vi "IMULoop.vi"(6 "I2CDevRef 2":T9={"DevStatus"={"status"=FALSE, "code"=0, "source"=""}, "Device Address"=0, "Handle"=0, "I2C Bus"=enum."Invalid"} {"Device Address" format="%.0x"}, 8 "AccelerometerDevRef":T1={"DevStatus"={"status"=FALSE, "code"=0, "source"=""}, "Scaling"={"Gain (VoltsPerG)"=0.0, "Center Voltage"=0.0}, "Analog Channels"={"X-Axis"=enum."Invalid", "Y-Axis"=enum."Invalid", "Z-Axis"=enum."Invalid"}, "I2C Bus"=enum."Invalid", "SPI Bus"=enum."Invalid", "Accel Range"=0, "ADXL345 Axes"={"X-Axis"=FALSE, "Y-Axis"=FALSE, "Z-Axis"=FALSE}, "Handle"=0, "Device Address"=0, "Accel Type"=enum."Analog"} {"Device Address" format="%.0x"; "Accel Range" items=["+/- 2 g", "+/- 4 g", "+/- 8 g", "+/- 16 g"]}) -> ()   [LabVIEW 2015]
uses:
  <vilib>/Rock Robotics/WPI/I2C/WPI_I2CDevRef.ctl
  <vilib>/Rock Robotics/SystemInterfaces/i2clib/i2c_bus.ctl
  <vilib>/Rock Robotics/WPI/Accelerometer/WPI_AccelerometerDevRef.ctl
  <vilib>/Rock Robotics/WPI/Accelerometer/WPI_AccelerometerScaling.ctl
  <vilib>/Rock Robotics/WPI/Accelerometer/WPI_AccelerometerAnalogChannels.ctl
  <vilib>/Rock Robotics/SystemInterfaces/AI/FPGA_AIChannel.ctl
  <vilib>/Rock Robotics/SystemInterfaces/spilib/spi_bus.ctl
  <vilib>/Rock Robotics/WPI/Accelerometer/ADXL345 Range.ctl
  <vilib>/Rock Robotics/WPI/Accelerometer/WPI_AccelerometerADXL345 Axes.ctl
  Common Code/IMU Data.ctl
  navX-MXP Library/COMMON/TypeDefs/Value TypeDefs/navX NAVX_CAL_STATUS.ctl
  navX-MXP Library/COMMON/TypeDefs/Value TypeDefs/navX NAVX_OP_STATUS.ctl
  Robot Global Data.vi
  <vilib>/Platform/TimedLoop/XDataNode/XDataNode.xnode
  <vilib>/Platform/TimedLoop/XDataNode/nitl_modes.ctl
  <vilib>/Platform/TimedLoop/XDataNode/XDNodeRunTimeDep.lvlib
  <vilib>/Platform/TimedLoop/XDataNode/wakeup.ctl
  <vilib>/Platform/TimedLoop/XDataNode/timing_clust.ctl
  navX-MXP Library/navX-MXP IMU.lvlib
panel:
  # "ADXL345"
  # "Analog"
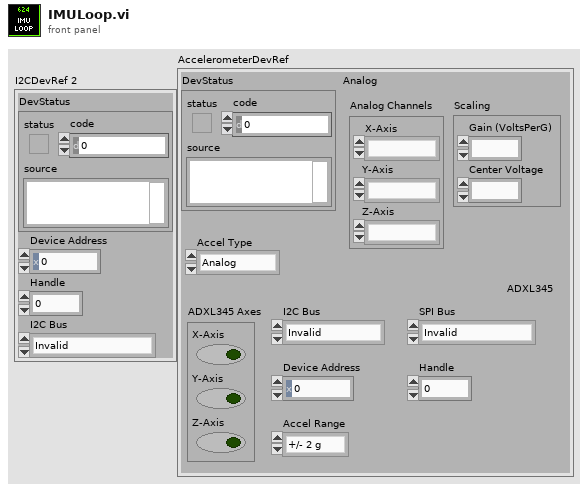
[diagram p1: front panel]
types:
  T1 = typedef "WPI_AccelerometerDevRef.ctl" = cluster{"DevStatus":errorcluster, "Scaling":T2, "Analog Channels":T3, "I2C Bus":T5, "SPI Bus":T6, "Accel Range":T7, "ADXL345 Axes":T8, "Handle":i32, "Device Address":u8, "Accel Type":enum16{"Analog", "ADXL345 I2C", "ADXL345 SPI", "Internal"}}
  T2 = typedef "WPI_AccelerometerScaling.ctl" = cluster{"Gain (VoltsPerG)":dbl, "Center Voltage":dbl}
  T3 = typedef "WPI_AccelerometerAnalogChannels.ctl" = cluster{"X-Axis":T4, "Y-Axis":T4, "Z-Axis":T4}
  T4 = typedef "FPGA_AIChannel.ctl" = enum8{"AI 0", "AI 1", "AI 2", "AI 3", "AI MXP 0", "AI MXP 1", "AI MXP 2", "AI MXP 3", "Invalid"}
  T5 = typedef "i2c_bus.ctl" = enum16{"I2C On-Board", "I2C MXP", "Invalid"}
  T6 = typedef "spi_bus.ctl" = enum16{"SPI On-Board, CS0", "SPI On-Board, CS1", "SPI On-Board, CS2", "SPI On-Board, CS3", "SPI MXP", "Invalid"}
  T7 = typedef "ADXL345 Range.ctl" = u8
  T8 = typedef "WPI_AccelerometerADXL345 Axes.ctl" = cluster{"X-Axis":bool, "Y-Axis":bool, "Z-Axis":bool}
  T9 = typedef "WPI_I2CDevRef.ctl" = cluster{"DevStatus":errorcluster, "Device Address":u8, "Handle":i32, "I2C Bus":T5}
  T10 = typedef "IMU Data.ctl" = cluster{"Pitch":sgl, "Roll":sgl, "Yaw":sgl, "Data Valid?":bool, "Temp":sgl, "MOVING":bool, "NAVX_CAL_STATUS":T11, "NAVX_OP_STATUS":T12, "YAW_STABLE":bool, "Accel X":sgl, "Accel Y":sgl, "Accel Z":sgl, "Accel Magnitude":sgl, "Pitch Rate":sgl, "Roll Rate":sgl, "Yaw Rate":sgl, "NavX Opened?":bool}
  T11 = typedef "navX-MXP IMU.lvlib/navX NAVX_CAL_STATUS.ctl" = u8
  T12 = typedef "navX-MXP IMU.lvlib/navX NAVX_OP_STATUS.ctl" = u8
  T13 = typedef "XDNodeRunTimeDep.lvlib/timing_clust.ctl" = cluster{"Expected End [f-1]":u64, "Actual End [f-1]":u64, "Finished Late? [f-1]":bool, "Expected End [i-1]":u64, "Actual End [i-1]":u64, "Finished Late? [i-1]":bool, "Expected Start [i]":u64, "Actual Start [i]":u64, "Expected Start [f]":u64, "Actual Start [f]":u64, "Source Name":string, "Structure Name":string, "Period":i64, "Deadline":i64, "Offset":i64, "Start":i64, "Priority":i32, "Timeout":i32, "Mode":T14, "Wakeup Reason":T15, "Error":errorcluster, "Source Type":string, "Secondary Source Type":string, "Global End Time":u64, "Global Start Time":u64, "Frame Duration":u64, "Iteration Duration":u64, "Assigned CPU":i32, "I/O Scan Engine Mode":u32}
  T14 = typedef "XDNodeRunTimeDep.lvlib/nitl_modes.ctl" = enum32{"No Change", "Process missed periods, maintain original phase", "Discard missed periods, maintain original phase", "Process missed periods, ignore original phase", "Discard missed periods, ignore original phase"}
  T15 = typedef "XDNodeRunTimeDep.lvlib/wakeup.ctl" = enum32{"Normal", "Aborted", "Asynchronous wakeup", "Timing source error", "Timed loop error", "Timeout"}
  T16 = cluster{"X-Axis":dbl, "Y-Axis":dbl, "Z-Axis":dbl}
  T17 = typedef "navX-MXP IMU.lvlib/navX Device TypeDef.ctl" = cluster{"navX Interface Protocol":T18, "navX Interface Protocol TypeDefs":cluster{"SPIDevRef":T19, "I2CDevRef":T9}, "navX System Information":cluster{"Board Information":T20, "Status":T21, "Offsets":T23}, "navX Common Information":cluster{"Update Rate (4Hz-60Hz)":T24, "refnum name":string, "error":errorcluster}}
  T18 = typedef "navX-MXP IMU.lvlib/navX Interface Protocol.ctl" = enum16{"SPI", "I2C"}
  T19 = typedef "WPI_SPIDevRef.ctl" = cluster{"DevStatus":errorcluster, "Handle":i32, "SPI Bus":T6}
  T20 = typedef "navX-MXP IMU.lvlib/navX Board Information.ctl" = cluster{"WhoAmI (50 | 0x32)":u8, "Board Revision":u8, "Firmware Major Version":u8, "Firmware Minor Version":u8}
  T21 = typedef "navX-MXP IMU.lvlib/navX Status Data.ctl" = cluster{"Update Rate Hz":u8, "Accelerometer Full-Scale Range":u8, "Gyro Full-Scale Range":u16, "NAVX_OP_STATUS":T12, "NAVX_CAL_STATUS":T11, "NAVX_SELFTEST_STATUS":u8, "NAVX_SENSOR_STATUS":T22}
  T22 = typedef "navX-MXP IMU.lvlib/navX NAVX_SENSOR_STATUS.ctl" = cluster{"MOVING":bool, "YAW_STABLE":bool, "MAG_DISTURBANCE":bool, "ALTITUDE_VALID":bool, "SEALEVEL_PRESS_SET":bool, "FUSED_HEADING_VALID":bool}
  T23 = typedef "navX-MXP IMU.lvlib/navX Offsets Data.ctl" = cluster{"Yaw":dbl, "Quat W":dbl, "Quat X":dbl, "Quat Y":dbl, "Quat Z":dbl}
  T24 = typedef "navX-MXP IMU.lvlib/navX Update Rate.ctl" = u8
  T25 = typedef "navX-MXP IMU.lvlib/navX Vector Data.ctl" = cluster{"X":dbl, "Y":dbl, "Z":dbl}
  T26 = typedef "navX-MXP IMU.lvlib/navX YPRH Data.ctl" = cluster{"Yaw":dbl, "Pitch":dbl, "Roll":dbl, "Heading":dbl}
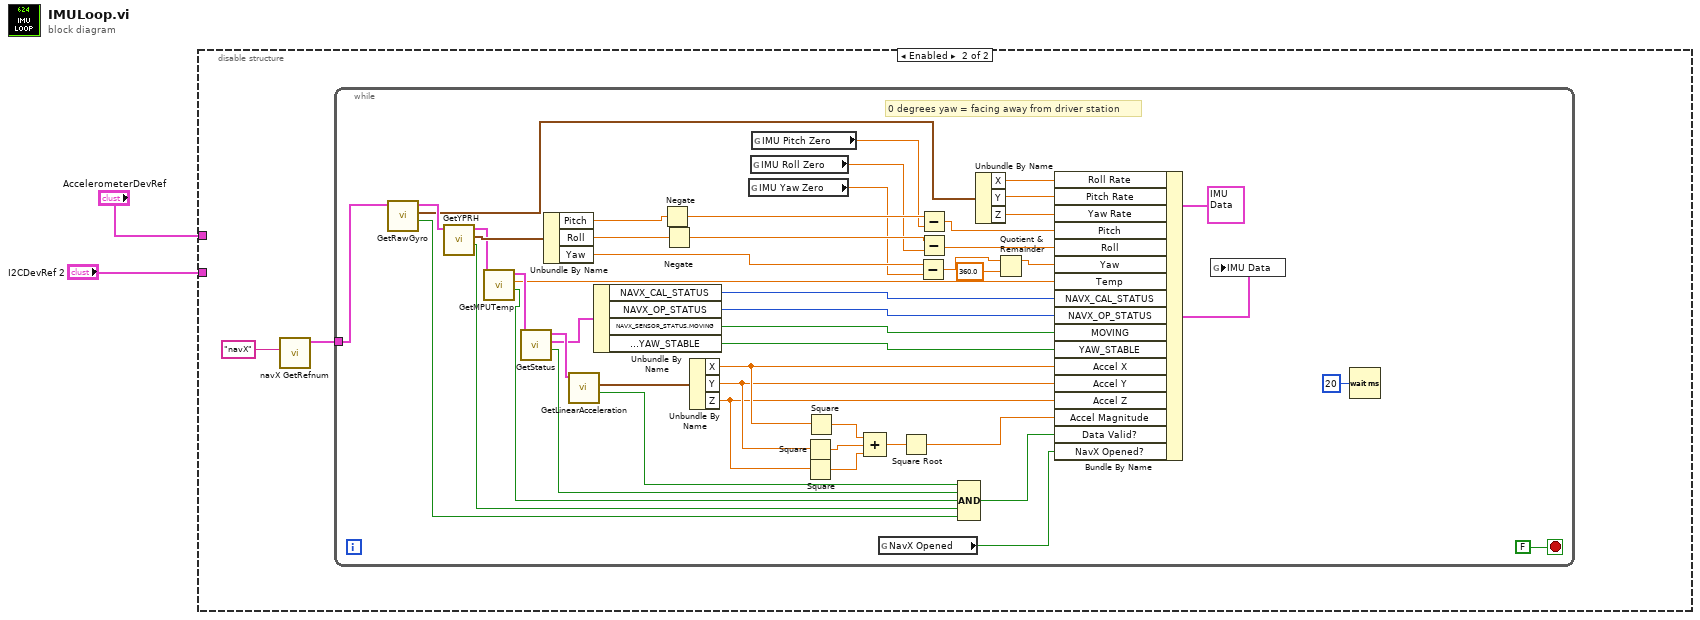
[diagram p0: block diagram]
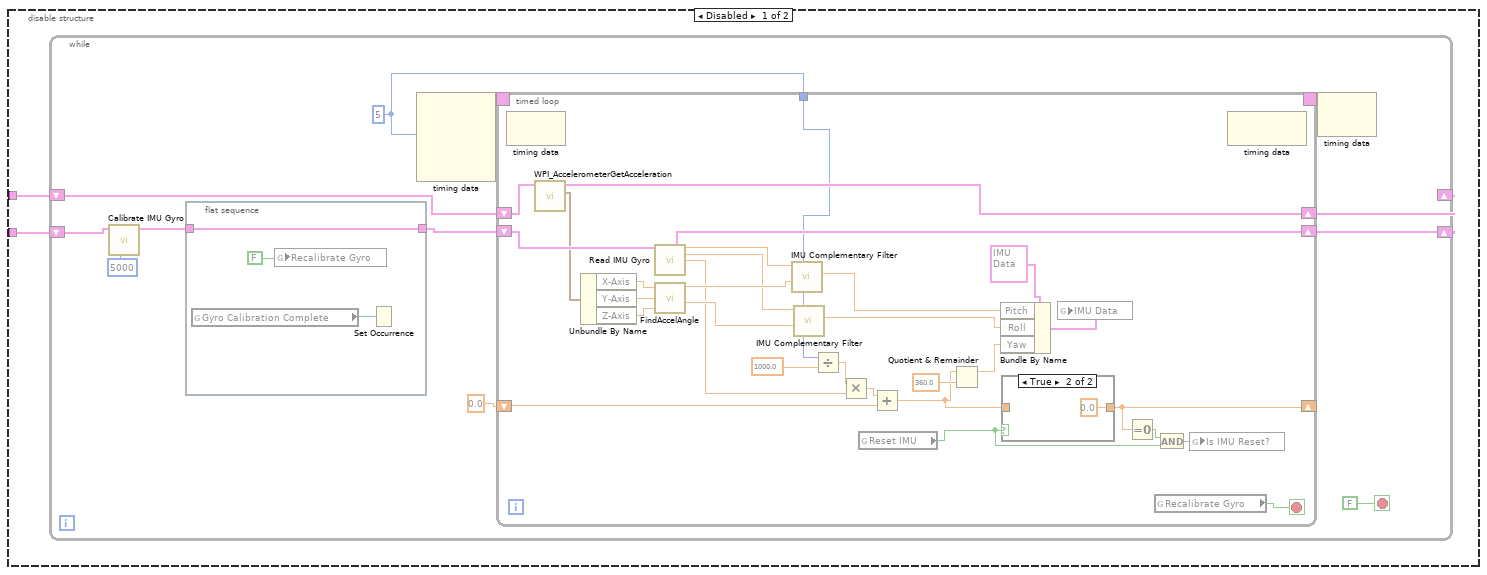
[diagram p2: hidden frame]
diagram:
  n1 = disable-structure shown="Enabled" {
    disable-tunnel: "I2CDevRef 2" -> [w4 _]
    disable-tunnel: "AccelerometerDevRef" -> [w3 _]
    frame Disabled {
      n2 = while {
        shift-right: [w9] -> _
        shift-left: w4 -> [w10]
        shift-right: [w8] -> _
        shift-left: w3 -> [w14]
        stop <- FALSE stop-if-true
        w13 = u16 5 ("Period")
        n3 = call "Calibrate IMU Gyro.vi"("Calib time (ms)"=u32 5000, "I2CDevRef in"=w10) -> ("I2CDevRef out"=w6:T9)  [unwired: 9 in]
        n4 = flat-sequence {
          tunnel: [w19] -> w5
          tunnel: w6 -> [w19]
          frame #0 {
            n5 = global read "Robot Global Data.vi" "Gyro Calibration Complete"() -> (w17:refnum<k4>)
            n6 = global write "Robot Global Data.vi" "Recalibrate Gyro"(FALSE ("Recalibrate Gyro")) -> ()
            n7 = Set Occurrence(w17) -> ()
          }
        }
        n8 = node-c288(w13) -> (w16:T13)  [unwired: 3 in]
        n9 = timed-loop {
          timing: w16 -> [_]
          timing-out: [_] -> w15
          shift-right: [w49] -> w9
          shift-left: w5 -> [w48]
          shift-right: [w46] -> w8
          shift-left: w14 -> [w47]
          tunnel: w13 -> [w44]
          shift-right: [w24] -> _
          shift-left: 0.0 -> [w45]
          stop <- w20 stop-if-true
          n10 = node-c288() -> ()  [unwired: 1 in, 1 out]
          n11 = call <vilib>:"WPI_AccelerometerGetAcceleration.vi"("AccelerometerDevRef"=w47) -> ("Accelerations"=w40:T16, "AccelerometerDevRef"=w46:T1)  [unwired: 8 in, 1 out]
          n12 = Unbundle By Name(w40) -> ("X-Axis"=w41:dbl, "Y-Axis"=w42:dbl, "Z-Axis"=w43:dbl)
          n13 = call "Read IMU Gyro.vi"("I2CDevRef"=w48) -> ("I2CDevRef 2"=w49:T9, "X"=w39:dbl, "Y"=w37:dbl, "Z"=w33:dbl)  [unwired: 8 in, 3 out]
          n14 = call "FindAccelAngle.vi"("Z"=w43, "Y"=w42, "X"=w41) -> ("Roll"=w36:dbl, "Pitch"=w38:dbl)  [unwired: 4 in]
          n15 = call "IMU Complementary Filter.vi"("dt (ms)"=w44, "Accelerometer Angle"=w38, "Angular vel (gyro, deg/sec)"=w39) -> ("Current Angle"=w28:dbl)  [unwired: 8 in]
          n16 = call "IMU Complementary Filter.vi"("dt (ms)"=w44, "Accelerometer Angle"=w36, "Angular vel (gyro, deg/sec)"=w37) -> ("Current Angle"=w29:dbl)  [unwired: 8 in]
          n17 = Divide(x=w44, y=1000.0) -> (x/y=w34:dbl)
          n18 = Multiply(x=w34, y=w33) -> (x*y=w32:dbl)
          n19 = global read "Robot Global Data.vi" "Reset IMU"() -> (w21:bool)
          n20 = Add(x=w32, y=w45) -> (x+y=w25:dbl)
          n21 = Quotient & Remainder(x=w25, y=360.0) -> (x-y*floor(x/y)=w26:dbl)  [unwired: 1 out]
          n22 = Bundle By Name(cluster=T10 {"Pitch"=0.0, "Roll"=0.0, "Yaw"=0.0, "Data Valid?"=FALSE, "Temp"=0.0, "MOVING"=FALSE, "NAVX_CAL_STATUS"=0, "NAVX_OP_STATUS"=0, "YAW_STABLE"=FALSE, "Accel X"=0.0, "Accel Y"=0.0, "Accel Z"=0.0, "Accel Magnitude"=0.0, "Pitch Rate"=0.0, "Roll Rate"=0.0, "Yaw Rate"=0.0, "NavX Opened?"=FALSE} ("IMU Data"), "Pitch"=w28, "Roll"=w29, "Yaw"=w26) -> (w30:T10)
          n23 = case shown="True" w21 {
            tunnel: w25 -> [w50 _]
            tunnel: [w50 0.0] -> w24
            frame False {
            }
            frame True {
            }
          }
          n24 = global write "Robot Global Data.vi" "IMU Data"(w30) -> ()
          n25 = Equal To 0?(x=w24) -> (x = 0?=w22:bool)
          n26 = global read "Robot Global Data.vi" "Recalibrate Gyro"() -> (w20:bool)
          n27 = And(x=w22, y=w21) -> (x .and. y?=w23:bool)
          n28 = global write "Robot Global Data.vi" "Is IMU Reset?"(w23) -> ()
          n29 = node-c288() -> ()  [unwired: 1 in, 1 out]
        }
        n30 = node-c288(w15) -> ()  [unwired: 1 out]
      }
    }
    frame Enabled {
      n31 = call "navX GetRefnum.vi"("refnum name"="navX") -> ("navX Device TypeDef"=w58:T17)  [unwired: 9 in, 1 out]
      n32 = while {
        tunnel: w58 -> [w66]
        stop <- FALSE stop-if-true
        # "0 degrees yaw = facing away from driver station"
        n33 = call "GetRawGyro.vi"("navX Device TypeDef"=w66) -> ("Valid?"=w64:bool, "Raw Gyro"=w65:T25, "navX Device TypeDef"=w67:T17)  [unwired: 8 in]
        n34 = call "GetYPRH.vi"("navX Device TypeDef"=w67) -> ("Valid?"=w83:bool, "YPRH"=w105:T26, "navX Device TypeDef"=w104:T17)  [unwired: 8 in]
        n35 = call "GetMPUTemp.vi"("navX Device TypeDef"=w104) -> ("Valid?"=w84:bool, "MPU Temperature (Centigrade)"=w100:dbl, "navX Device TypeDef"=w103:T17)  [unwired: 8 in]
        n36 = call "GetStatus.vi"("navX Device TypeDef"=w103) -> ("Valid?"=w85:bool, "Status"=w101:T21, "navX Device TypeDef"=w102:T17)  [unwired: 8 in]
        n37 = Unbundle By Name(w105) -> ("Pitch"=w80:dbl, "Roll"=w79:dbl, "Yaw"=w69:dbl)
        n38 = call "GetLinearAcceleration.vi"("navX Device TypeDef"=w102) -> ("Valid?"=w86:bool, "Linear Acceleration"=w95:T25)  [unwired: 8 in, 1 out]
        n39 = Unbundle By Name(w101) -> ("NAVX_CAL_STATUS"=w99:T11, "NAVX_OP_STATUS"=w98:T12, "NAVX_SENSOR_STATUS.MOVING"=w97:bool, "NAVX_SENSOR_STATUS.YAW_STABLE"=w96:bool)
        n40 = Negate(x=w80) -> (-x=w77:dbl)
        n41 = Negate(x=w79) -> (-x=w75:dbl)
        n42 = Unbundle By Name(w95) -> ("X"=w94:dbl, "Y"=w93:dbl, "Z"=w92:dbl)
        n43 = global read "Robot Global Data.vi" "IMU Yaw Zero"() -> (w68:dbl)
        n44 = global read "Robot Global Data.vi" "IMU Roll Zero"() -> (w74:dbl)
        n45 = global read "Robot Global Data.vi" "IMU Pitch Zero"() -> (w76:dbl)
        n46 = Square(x=w93) -> (x^2=w90:dbl)
        n47 = Square(x=w92) -> (x^2=w89:dbl)
        n48 = Square(x=w94) -> (x^2=w91:dbl)
        n49 = Compound Arithmetic op=ADD(w91, w90, w89) -> (w88:dbl)
        n50 = global read "Robot Global Data.vi" "NavX Opened"() -> (w60:bool)
        n51 = Square Root(x=w88) -> (sqrt(x)=w87:dbl)
        n52 = Subtract(x=w69, y=w68) -> (x-y=w70:dbl)
        n53 = Subtract(x=w77, y=w76) -> (x-y=w73:dbl)
        n54 = Subtract(x=w75, y=w74) -> (x-y=w72:dbl)
        n55 = Compound Arithmetic op=AND(w86, w85, w84, w83, w64) -> (w82:bool)
        n56 = Unbundle By Name(w65) -> ("X"=w62:dbl, "Y"=w61:dbl, "Z"=w63:dbl)
        n57 = Quotient & Remainder(x=w70, y=360.0) -> (x-y*floor(x/y)=w71:dbl)  [unwired: 1 out]
        n58 = Bundle By Name(cluster=T10 {"Pitch"=0.0, "Roll"=0.0, "Yaw"=0.0, "Data Valid?"=FALSE, "Temp"=0.0, "MOVING"=FALSE, "NAVX_CAL_STATUS"=0, "NAVX_OP_STATUS"=0, "YAW_STABLE"=FALSE, "Accel X"=0.0, "Accel Y"=0.0, "Accel Z"=0.0, "Accel Magnitude"=0.0, "Pitch Rate"=0.0, "Roll Rate"=0.0, "Yaw Rate"=0.0, "NavX Opened?"=FALSE} ("IMU Data"), "Roll Rate"=w62, "Pitch Rate"=w61, "Yaw Rate"=w63, "Pitch"=w73, "Roll"=w72, "Yaw"=w71, "Temp"=w100, "NAVX_CAL_STATUS"=w99, "NAVX_OP_STATUS"=w98, "MOVING"=w97, "YAW_STABLE"=w96, "Accel X"=w94, "Accel Y"=w93, "Accel Z"=w92, "Accel Magnitude"=w87, "Data Valid?"=w82, "NavX Opened?"=w60) -> (w106:T10)
        n59 = global write "Robot Global Data.vi" "IMU Data"(w106) -> ()
        n60 = Wait (ms)(milliseconds to wait=u32 20) -> ()  [unwired: 1 out]
      }
    }
  }
